vi "sv_Swept Integration Time to Samples.vi"(6 "integration time":T2 {"integration time" format="%.2f"}, 7 "frequency to generate [Hz]":dbl format="%.2f", 10 "AI sampling frequency":dbl format="%.2f", 11 "indice computations in":T1) -> (2 "dup AI sampling frequency":dbl format="%.2f", 3 "indice computations in":T1)   [LabVIEW 2017, in "SoundVib_SweptSine.lvlib"]
uses:
  <vilib>/addons/Sound and Vibration/svt_Swept Sine/SoundVib_SweptSine.lvlib
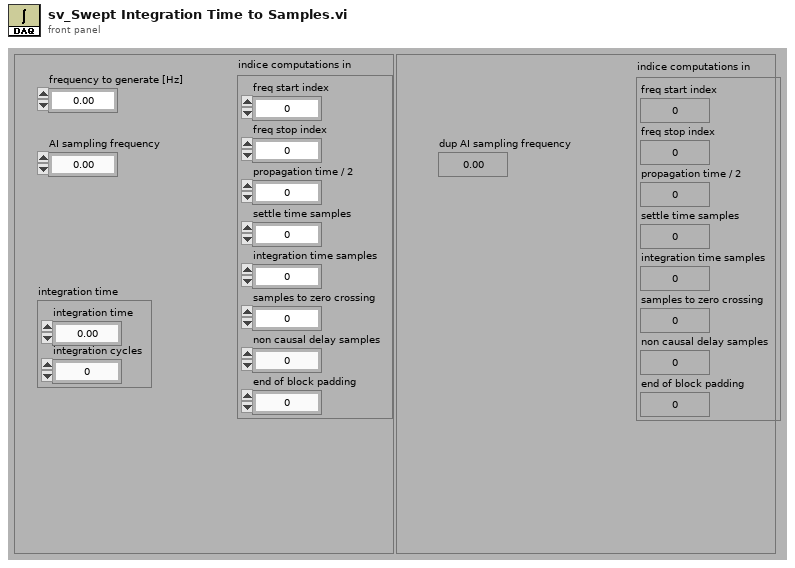
[diagram p1: front panel]
types:
  T1 = cluster{"freq start index":u32, "freq stop index":u32, "propagation time / 2":u32, "settle time samples":u32, "integration time samples":u32, "samples to zero crossing":u32, "non causal delay samples":u32, "end of block padding":u32}
  T2 = cluster{"integration time":dbl, "integration cycles":i32}
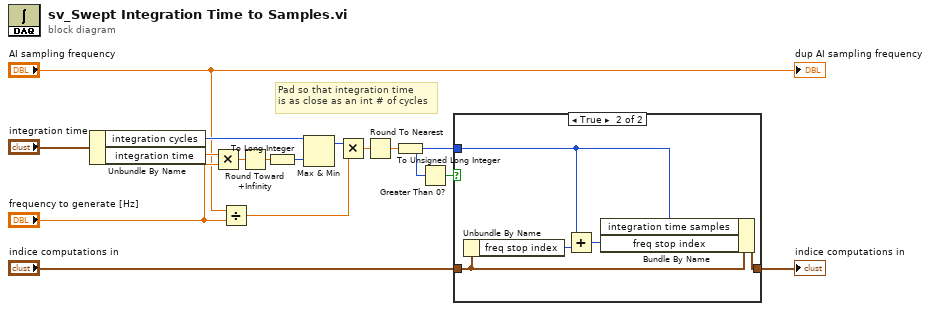
[diagram p0: block diagram]
diagram:
  # "Pad so that integration time \nis as close as an int # of cycles"
  n1 = Unbundle By Name("integration time") -> ("integration cycles"=w7:i32, "integration time"=w6:dbl)
  n2 = Multiply(x=w6, y="frequency to generate [Hz]") -> (x*y=w14:dbl)
  n3 = Divide(x="AI sampling frequency", y="frequency to generate [Hz]") -> (x/y=w9:dbl)
  n4 = Round Toward +Infinity(x=w14) -> (ceil(x): smallest int >= x=w13:dbl)
  n5 = To Long Integer(number=w13) -> (32bit integer=w12:i32)
  n6 = Max & Min(x=w7, y=w12) -> (max(x,y)=w10:i32)  [unwired: 1 out]
  n7 = Multiply(x=w10, y=w9) -> (x*y=w11:dbl)
  n8 = Round To Nearest(number=w11) -> (nearest integer value=w15:dbl)
  n9 = To Unsigned Long Integer(number=w15) -> (unsigned 32bit integer=w2:u32)
  n10 = Greater Than 0?(x=w2) -> (x > 0?=w3:bool)
  n11 = case shown="True" w3 {
    tunnel: w2 -> [_ w20]
    tunnel: "indice computations in" -> [w17 w19]
    tunnel: [w17 w18] -> w1
    frame False {
    }
    frame True {
      n12 = Unbundle By Name(w19) -> ("freq stop index"=w21:u32)
      n13 = Add(x=w20, y=w21) -> (x+y=w22:u32)
      n14 = Bundle By Name(cluster=w19, "integration time samples"=w20, "freq stop index"=w22) -> (w18:T1)
    }
  }
  "indice computations in" <- w1
  "dup AI sampling frequency" <- "AI sampling frequency"
